vi "sample0(Basic).vi"   [LabVIEW 2011]
types:
  T1 = cluster{"XM/XH Address":u16, "size":u16, cluster{"id":u8, "array":u8[]}[]}
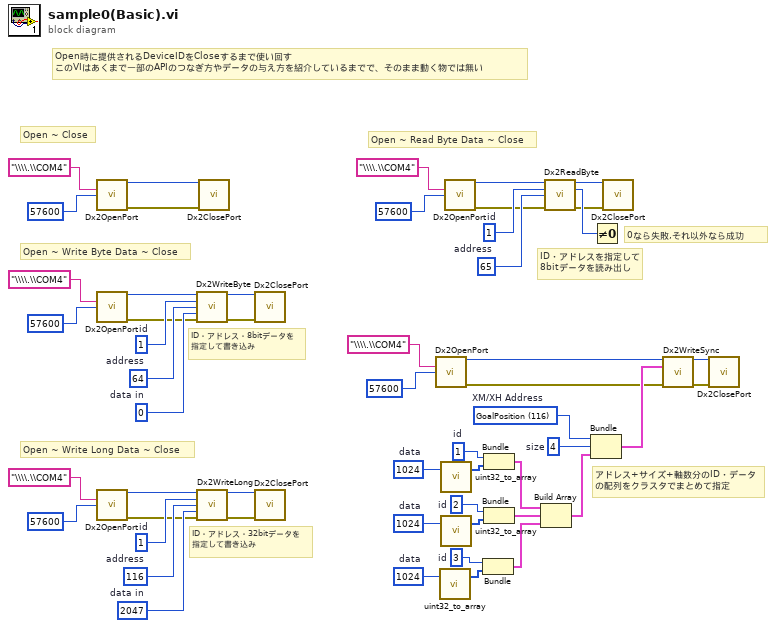
[diagram p0: block diagram]
diagram:
  w12 = u8 1  # id
  w13 = u8 3  # id
  w14 = u8 2  # id
  w17 = 1024  # data
  w16 = 1024  # data
  w15 = 1024  # data
  w20 = u16 116 items=["ModelNo"=0, "ModelInfo"=2, "VersionOfFirmware"=6, "ID"=7, "Baudrate"=8, "ReturnDelayTime"=9, "OperationMode"=11, "ProtocolVersion"=13, "HormingOffset"=20, "MovingThreshold"=24, "TemperatureLimit"=31, "MaxVoltageLimit"=32, "MinVoltageLimit"=34, "PWMLimit"=36, "CurrentLimit"=38, "AccelerationLimit"=40, "VelocityLimit"=44, "MaxPositionLimit"=48, "MinPositionLimit"=52, "Shutdown"=63, "TorqueEnable"=64, "LED"=65, "StatusReturnLevel"=68, "RegistedInstruction"=69, "HardwareErrorStatus"=70, "VelocityIGain"=76, "VelocityPGain"=78, "VelocityDGain"=80, "PositionIGain"=82, "PositionPGain"=84, "FeedForward2ndGain"=88, "FeedForward1stGain"=90, "GoalPWM"=100, "GoalCurrent"=102, "GoalVelocity"=104, "ProfileAcceleration"=108, "ProfileVelocity"=112, "GoalPosition"=116, "RealtimeTick"=120, "Moving"=122, "MovingStatus"=123, "PresentPWM"=124, "PresentCurrent"=126, "Presentvelocity"=128, "PresentPosition"=132, "VelocityTrajectory"=136, "PositionTrajectory"=140, "PresentIInputVoltage"=144, "PresentTemperature"=146]  # XM/XH Address
  w29 = u16 4  # size
  w34 = u16 65  # address
  w33 = u8 1  # id
  w41 = u32 2047  # data in
  w40 = u16 116  # address
  w39 = u8 1  # id
  w46 = u8 0  # data in
  w47 = u16 64  # address
  w48 = u8 1  # id
  # "0なら失敗,それ以外なら成功"
  # "ID・アドレスを指定して\n8bitデータを読み出し"
  # "ID・アドレス・8bitデータを\n指定して書き込み"
  # "ID・アドレス・32bitデータを\n指定して書き込み"
  # "アドレス+サイズ+軸数分のID・データ\nの配列をクラスタでまとめて指定"
  # "Open ~ Read Byte Data ~ Close"
  # "Open ~ Write Long Data ~ Close"
  # "Open ~ Write Byte Data ~ Close"
  # "Open ~ Close"
  # "Open時に提供されるDeviceIDをCloseするまで使い回す\nこのVIはあくまで一部のAPIのつなぎ方やデータの与え方を紹介しているまでで、そのまま動く物では無い"
  n1 = call "Dx2OpenPort.vi"("port"="\\\\.\\COM4", "baudrate"=u32 57600) -> ("dvid"=w51:u32, "エラー出力"=w9:errorcluster)  [unwired: 11 in, 1 out]
  n2 = call "Dx2OpenPort.vi"("port"="\\\\.\\COM4", "baudrate"=u32 57600) -> ("dvid"=w49:u32, "エラー出力"=w8:errorcluster)  [unwired: 11 in, 1 out]
  n3 = call "Dx2OpenPort.vi"("port"="\\\\.\\COM4", "baudrate"=u32 57600) -> ("dvid"=w38:u32, "エラー出力"=w6:errorcluster)  [unwired: 11 in, 1 out]
  n4 = call "Dx2WriteByte.vi"("dvid in"=w49, "id"=w48, "address"=w47, "data in"=w46, "エラー入力"=w8) -> ("dvid out"=w44:u32, "エラー出力"=w7:errorcluster)  [unwired: 8 in, 1 out]
  n5 = call "Dx2WriteLong.vi"("dvid in"=w38, "id"=w39, "address"=w40, "data in"=w41, "エラー入力"=w6) -> ("dvid out"=w43:u32, "エラー出力"=w5:errorcluster)  [unwired: 8 in, 1 out]
  n6 = call "Dx2ClosePort.vi"("dvid"=w51, "エラー入力"=w9) -> ()  [unwired: 12 in, 2 out]
  n7 = call "Dx2ClosePort.vi"("dvid"=w44, "エラー入力"=w7) -> ()  [unwired: 12 in, 2 out]
  n8 = call "Dx2ClosePort.vi"("dvid"=w43, "エラー入力"=w5) -> ()  [unwired: 12 in, 2 out]
  n9 = call "Dx2OpenPort.vi"("port"="\\\\.\\COM4", "baudrate"=u32 57600) -> ("dvid"=w11:u32, "エラー出力"=w2:errorcluster)  [unwired: 11 in, 1 out]
  n10 = call "uint32_to_array.vi"("uint32"=w17) -> ("array"=w27:u8[])  [unwired: 2 in]
  n11 = call "uint32_to_array.vi"("uint32"=w15) -> ("array"=w28:u8[])  [unwired: 2 in]
  n12 = call "uint32_to_array.vi"("uint32"=w16) -> ("array"=w26:u8[])  [unwired: 2 in]
  n13 = call "Dx2OpenPort.vi"("port"="\\\\.\\COM4", "baudrate"=u32 57600) -> ("dvid"=w32:u32, "エラー出力"=w4:errorcluster)  [unwired: 11 in, 1 out]
  n14 = Bundle("id"=w13, "array"=w27) -> (w24:cluster{"id":u8, "array":u8[]})  [unwired: 1 in]
  n15 = Bundle("id"=w12, "array"=w28) -> (w23:cluster{"id":u8, "array":u8[]})  [unwired: 1 in]
  n16 = Bundle("id"=w14, "array"=w26) -> (w25:cluster{"id":u8, "array":u8[]})  [unwired: 1 in]
  n17 = Build Array(w23, w25, w24) -> (w22:cluster{"id":u8, "array":u8[]}[])
  n18 = call "Dx2ReadByte.vi"("dvid in"=w32, "id"=w33, "address"=w34, "エラー入力"=w4) -> ("dvid out"=w36:u32, "data out"=w30:u8, "エラー出力"=w3:errorcluster)  [unwired: 8 in, 1 out]
  n19 = Bundle("XM/XH Address"=w20, "size"=w29, w22) -> (w21:T1)  [unwired: 1 in]
  n20 = Not Equal To 0?(x=w30) -> ()  [unwired: 1 out]
  n21 = call "Dx2ClosePort.vi"("dvid"=w36, "エラー入力"=w3) -> ()  [unwired: 12 in, 2 out]
  n22 = call "Dx2WriteSync.vi"("dvid in"=w11, "data in"=w21, "エラー入力"=w2) -> ("dvid out"=w10:u32, "エラー出力"=w1:errorcluster)  [unwired: 10 in, 1 out]
  n23 = call "Dx2ClosePort.vi"("dvid"=w10, "エラー入力"=w1) -> ()  [unwired: 12 in, 2 out]
